vi "LAUNCHER.vi"() -> ()   [LabVIEW 2019]
uses:
  UI_PAPAS_USD_ESP/UI_PAPAS_USD_ESP.lvclass
  C:/Program Files (x86)/National Instruments/LabVIEW 2019/vi.lib/ActorFramework/Actor/Actor.lvclass
  UI_PAPAS_MEX_ESP/UI_PAPAS_MEX_ESP.lvclass
  <vilib>/ActorFramework/Actor/Actor.lvclass
panel:
  in  "ABRIR":bool
  in  "stop":bool
  in  "IDIOMA":enum16{"INGLÉS", "ESPAÑOL"}(ring)
  in  "TIPO DE MONEDA":enum16{"USD", "MXN"}(ring)
  in  "PRODUCTO":enum16{"FRITURAS", "CAFÉ"}(ring)
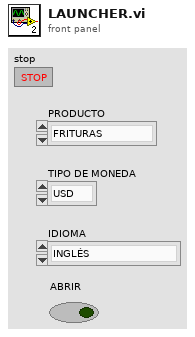
[diagram p1: front panel]
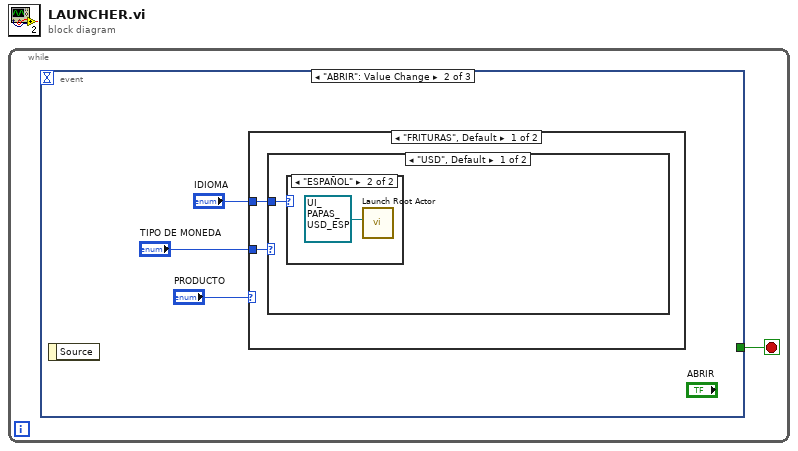
[diagram p0: block diagram]
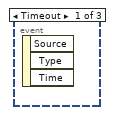
[diagram p2: hidden frame]
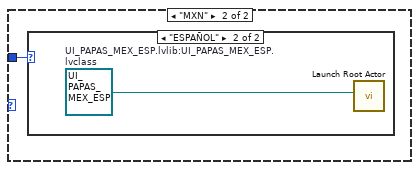
[diagram p4: hidden frame]
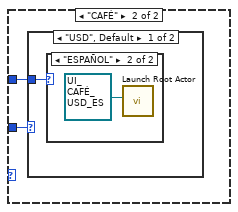
[diagram p6: hidden frame]
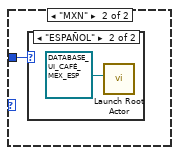
[diagram p8: hidden frame]
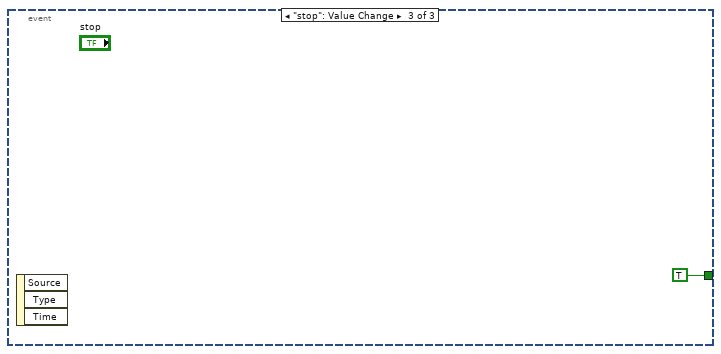
[diagram p10: hidden frame]
diagram:
  n1 = while {
    stop <- w1 stop-if-true
    n2 = event shown="[1] \"ABRIR\": Value Change" {
      selector: _ -> [_ _ _]
      dyn-events: _ -> [_ _ _]
      timeout: _ -> [_ _ _]
      tunnel: [_ _ TRUE] -> w1
      event Timeout {
        n3 = event-data() -> ()  [unwired: 1 in, 3 out]
      }
      event "ABRIR": Value Change {
        n4 = event-data() -> ()  [unwired: 1 in, 1 out]
        n5 = case shown="\"FRITURAS\", Default" "PRODUCTO" {
          tunnel: "TIPO DE MONEDA" -> [w6 w12]
          tunnel: "IDIOMA" -> [w5 w11]
          frame "FRITURAS", Default {
            n6 = case shown="\"USD\", Default" w6 {
              tunnel: w5 -> [w7 w9]
              frame "USD", Default {
                n7 = case shown="\"ESPAÑOL\"" w7 {
                  frame "INGLÉS", Default {
                  }
                  frame "ESPAÑOL" {
                    n8 = call <vilib>:"Launch Root Actor.vi"("Actor"=refnum<class "UI_PAPAS_USD_ESP.lvclass"> refnum ("UI_PAPAS_USD_ESP.lvlib:UI_PAPAS_USD_ESP.lvclass")) -> ()  [unwired: 9 in, 2 out]
                  }
                }
              }
              frame "MXN" {
                n9 = case shown="\"ESPAÑOL\"" w9 {
                  frame "INGLÉS", Default {
                  }
                  frame "ESPAÑOL" {
                    w10 = refnum<class "UI_PAPAS_MEX_ESP.lvclass"> refnum  # UI_PAPAS_MEX_ESP.lvlib:UI_PAPAS_MEX_ESP.lvclass
                    n10 = call <vilib>:"Launch Root Actor.vi"("Actor"=w10) -> ()  [unwired: 9 in, 2 out]
                  }
                }
              }
            }
          }
          frame "CAFÉ" {
            n11 = case shown="\"USD\", Default" w12 {
              tunnel: w11 -> [w13 w15]
              frame "USD", Default {
                n12 = case shown="\"ESPAÑOL\"" w13 {
                  frame "INGLÉS", Default {
                  }
                  frame "ESPAÑOL" {
                    n13 = call <vilib>:"Launch Root Actor.vi"("Actor"=refnum<class "UI_CAFÉ_USD_ES.lvclass"> refnum ("UI_CAFÉ_USD_ES.lvlib:UI_CAFÉ_USD_ES.lvclass")) -> ()  [unwired: 9 in, 2 out]
                  }
                }
              }
              frame "MXN" {
                n14 = case shown="\"ESPAÑOL\"" w15 {
                  frame "INGLÉS", Default {
                  }
                  frame "ESPAÑOL" {
                    n15 = call <vilib>:"Launch Root Actor.vi"("Actor"=refnum<class "DATABASE_UI_CAFÉ_MEX_ESP.lvclass"> refnum ("D_UI_CAFÉ_MEX_ESP.lvlib:DATABASE_UI_CAFÉ_MEX_ESP.lvclass")) -> ()  [unwired: 9 in, 2 out]
                  }
                }
              }
            }
          }
        }
      }
      event "stop": Value Change {
        n16 = event-data() -> ()  [unwired: 1 in, 3 out]
      }
    }
  }
